vi "Get Column Timestamp.vi"(8 "error in (no error)":errorcluster, 11 "PQ Result  in":refnum<class "PQ Result.lvclass">) -> (0 "error out":errorcluster, 2 "Timestamp":timestamp, 3 "PQ Result  out":refnum<class "PQ Result.lvclass">)   [LabVIEW 2013, in "PQ Result.lvclass"]
uses:
  PQ Result.lvclass
  Support/PQ Support.lvlib
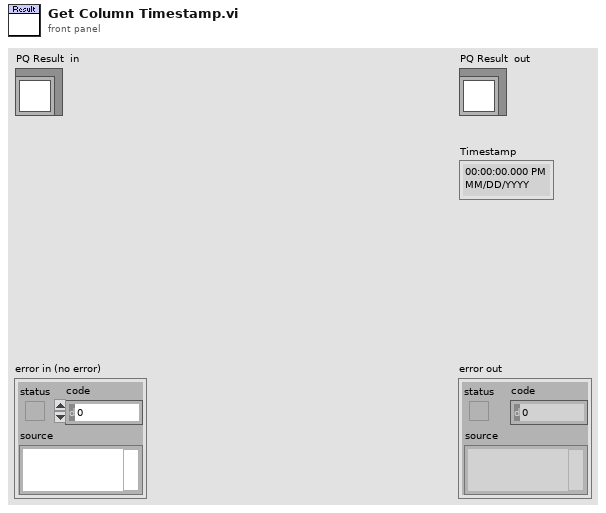
[diagram p1: front panel]
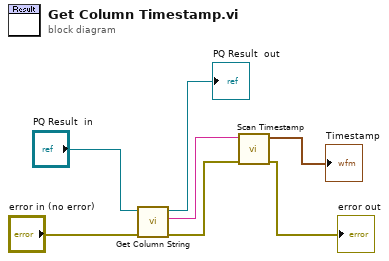
[diagram p0: block diagram]
diagram:
  n1 = call "Get Column String.vi"("error in (no error)"="error in (no error)", "PQ Result  in"="PQ Result  in") -> ("error out"=w2:errorcluster, "String"=w4:string, "PQ Result  out"=→"PQ Result  out":refnum<class "PQ Result.lvclass">)  [unwired: 7 in]
  n2 = call "Scan Timestamp.vi"("error in (no error)"=w2, "String"=w4) -> ("error out"=→"error out":errorcluster, "Timestamp"=→"Timestamp":timestamp)  [unwired: 8 in]
